vi "Keys.vi"(7 "array in":T1) -> (2 "keys":string[](array[string]), 3 "duplicate array":T1)   [LabVIEW 2015, in "Car Wash.lvlib" / "Tools_KeyedArray.lvlib"]
doc: "Returns an array containing the keys of all the elements in <B>array in</B>."
uses:
  Tools_KeyedArray.lvlib
  KeyedArray.ctl
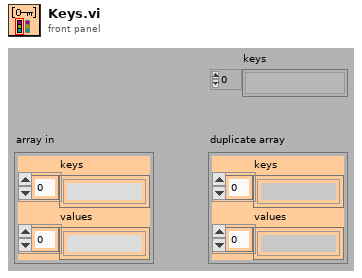
[diagram p1: front panel]
types:
  T1 = typedef "Car Wash.lvlib/Tools_KeyedArray.lvlib/KeyedArray.ctl" = cluster{"keys":string[], "values":string[]}
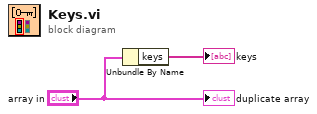
[diagram p0: block diagram]
diagram:
  n1 = Unbundle By Name("array in") -> ("keys"=→"keys":string[])
  "duplicate array" <- "array in"
